vi "Ctor.vi"(8 "error in (no error)":errorcluster, 10 "Baud (9600)":u32=9600, 11 "VISA Port":refnum<visa-resource-name>) -> (0 "error out":errorcluster, 3 "VISA GPS out":refnum<class "VISA GPS.lvclass">)   [LabVIEW 2020, in "nmea.lvlib" / "VISA GPS.lvclass"]
uses:
  VISA GPS.lvclass
  Ref Data.ctl
  VISA GPS.lvclass/VISA GPS.ctl
  <vilib>/Instr/_visa.llb/VISA Configure Serial Port (Instr).vi
  nmea/nmea.lvclass
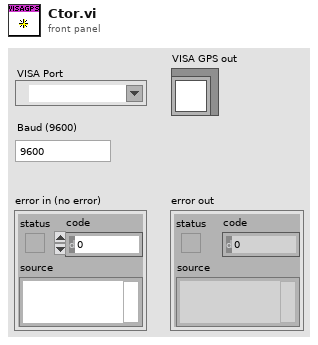
[diagram p1: front panel]
types:
  T1 = typedef "nmea.lvlib/VISA GPS.lvclass/Ref Data.ctl" = cluster{"Close":bool}
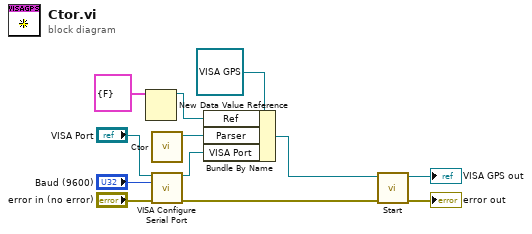
[diagram p0: block diagram]
diagram:
  n1 = New Data Value Reference(data value=T1 {"Close"=FALSE} ("Ref Data")) -> (data value reference=w10:refnum<data-value>)  [unwired: 1 in, 1 out]
  n2 = call "Ctor.vi"() -> ("nmea out"=w9:refnum<class "nmea.lvclass">)  [unwired: 10 in, 1 out]
  n3 = call-poly "VISA Configure Serial Port"("VISA resource name"="VISA Port", "baud rate (9600)"="Baud (9600)", "error in (no error)"="error in (no error)") -> ("VISA resource name out"=w1:refnum<visa-resource-name>, "error out"=w2:errorcluster)  [unwired: 11 in]
  n4 = Bundle By Name(cluster=refnum<class "VISA GPS.lvclass"> refnum ("VISA GPS in"), "Ref"=w10, "Parser"=w9, "VISA Port"=w1) -> (w8:refnum<class "VISA GPS.lvclass">)
  n5 = call "Start.vi"("error in (no error)"=w2, "VISA GPS in"=w8) -> ("error out"=→"error out":errorcluster, "VISA GPS out"=→"VISA GPS out":refnum<class "VISA GPS.lvclass">)  [unwired: 8 in]
